vi "midi_open_with_user_event.vi"(8 "error in (no error)":errorcluster, 9 "MidiData":refnum<user-event>, 10 "device_id":i32, 11 "LabVIEW-MIDI-XPLAT in":refnum<class "LabVIEW-MIDI-XPLAT.lvclass">) -> (0 "error out":errorcluster, 2 "Return":i32, 3 "LabVIEW-MIDI-XPLAT out":refnum<class "LabVIEW-MIDI-XPLAT.lvclass">)   [LabVIEW 2020, in "LabVIEW-MIDI-XPLAT.lvclass"]
uses:
  LabVIEW-MIDI-XPLAT.lvclass
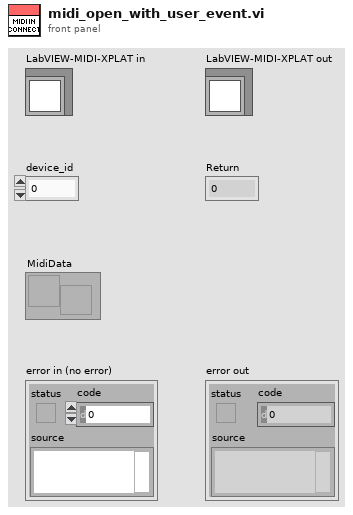
[diagram p1: front panel]
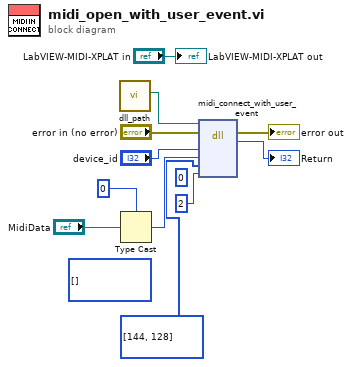
[diagram p0: block diagram]
diagram:
  (unwired) u8[] [] ("filter_array")
  (unwired) 0 ("array_size")
  n1 = call "dll_path.vi"() -> ("dll"=w7:path)  [unwired: 11 in]
  n2 = Type Cast(type=u32 0, x="MidiData") -> (*(type *) &x=w6:u32)
  n3 = dll-call lib="C:/code/LabVIEW-MIDI-XPLAT/dist/TomMIDIllan_*.*" fn="midi_connect_with_user_event"(path in=w7, error in="error in (no error)", "device_id"="device_id", "user_event_ref"=w6, "filter_array"=u8[] [144, 128], "array_size"=2) -> (error out=→"error out":errorcluster, "handle"=→"Return":i32)  [unwired: 5 in, 1 out]
  "LabVIEW-MIDI-XPLAT out" <- "LabVIEW-MIDI-XPLAT in"
